vi "Model Initial Values - Remove Inport RTM.vi"(8 "error in (no error)":errorcluster, 11 "Node Ptr":u64 format="%.0x") -> (0 "error out":errorcluster)   [LabVIEW 2011, in "Model Initial Values Custom Device.lvlib"]
uses:
  Model Initial Values Custom Device.lvlib
  <vilib>/NI Veristand/Custom Device API/Custom Device Item Ref.ctl
  NationalInstruments.VeriStand.SystemStorage
  Model Initial Values - Global.vi
  <vilib>/NI Veristand/Custom Device API/Get Item Property (Dependent Node Pointer).vi
  <vilib>/NI Veristand/Custom Device API/Set Item Property (Double Array).vi
  <vilib>/NI Veristand/Custom Device API/Set Item Property (String Array).vi
  <vilib>/NI Veristand/Custom Device Tools/Custom Device Utility Library/Custom Device Utility Library.lvlib
  <vilib>/NI Veristand/Custom Device API/Custom Device API.lvlib
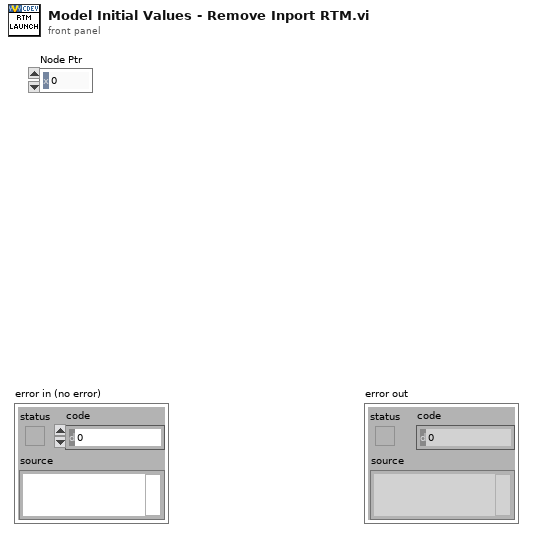
[diagram p1: front panel]
types:
  T1 = typedef "Custom Device API.lvlib/Custom Device Item Ref.ctl" = u64
  T2 = cluster{"MultipleSelection":bool, "ShowCheckBox":bool}
  T3 = typedef "Custom Device API.lvlib/Custom Device Item Info.ctl" = cluster{"Name":string, "Is Channel":bool, "GUID":string}
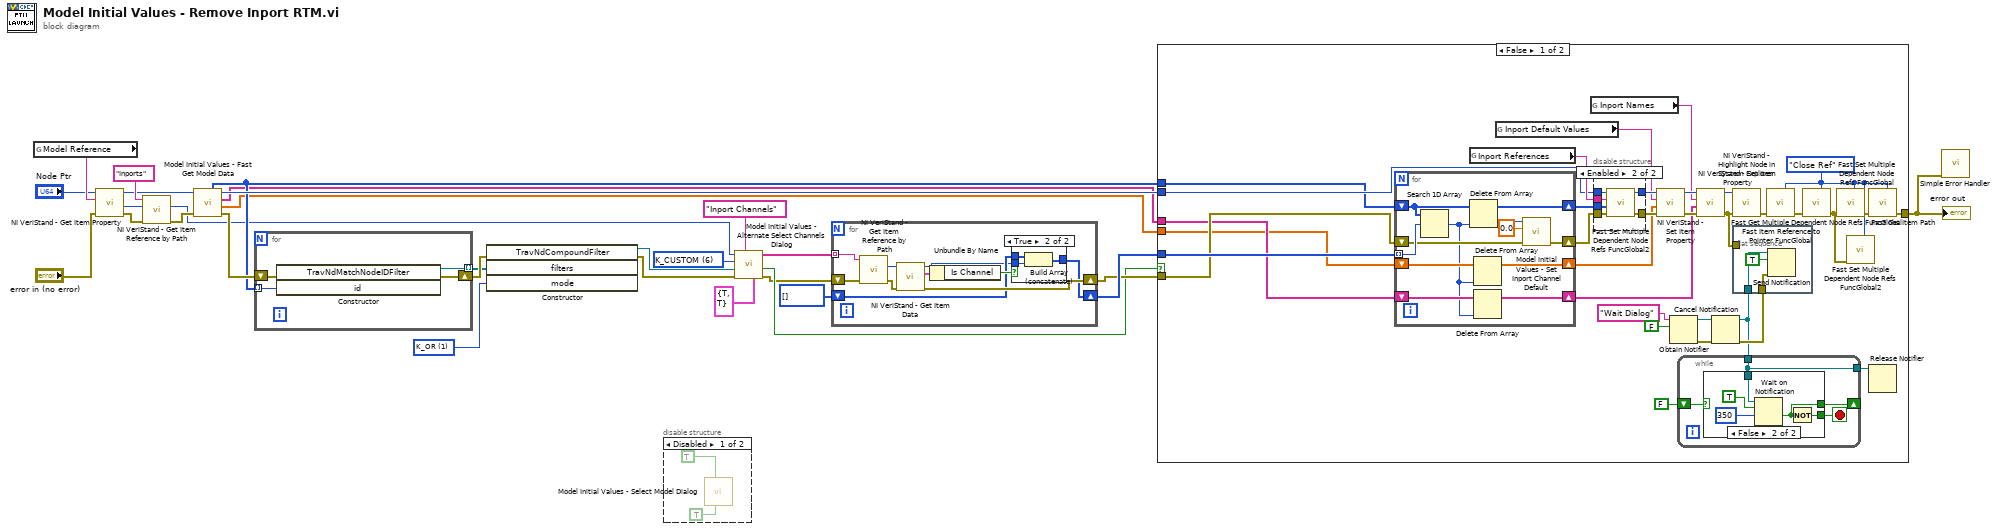
[diagram p0: block diagram]
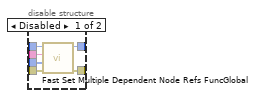
[diagram p4: hidden frame]
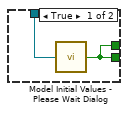
[diagram p5: hidden frame]
diagram:
  w13 = 1 items=["K_AND", "K_OR"] ("mode")
  w18 = u8 6 items=["K_CHAN_R", "K_CHAN_W", "K_CHAN_RW", "K_CHAN_VOLT", "K_CHAN_FAULT", "K_ALL", "K_CUSTOM"] ("Filter")
  n1 = global read "Model Initial Values - Global.vi" "Model Reference"() -> (w9:string)
  n2 = call-poly <vilib>:"NI VeriStand - Get Item Property.vi"("error in (no error)"="error in (no error)", "Property Name"=w9, "Item Ref in"="Node Ptr") -> ("error out"=w3:errorcluster, "Dependent Node Ref"=w4:T1, "Item Ref out"=w6:T1)  [unwired: 5 in, 1 out]
  n3 = call <vilib>:"NI VeriStand - Get Item Reference by Path.vi"("error in (no error)"=w3, "Root Ref"=w4, "Item Path in"="Inports" ("Relative Item Path")) -> ("error out"=w2:errorcluster, "Item Ref"=w1:T1)  [unwired: 5 in, 2 out]
  n4 = call "Model Initial Values - Fast Get Model Data.vi"("error in (no error)"=w2, "Local Model Ref in"=w6) -> ("error out"=w24:errorcluster, "Inport Default Values"=w21:dbl[], "Inport Names"=w22:string[], "Local Model Ref out"=w25:T1, "Inport Refs"=w23:T1[])  [unwired: 4 in, 1 out]
  n5 = for {
    tunnel: [w33] -> w12 mode=indexing
    shift-right: [w32] -> w14
    shift-left: w24 -> [w31]
    tunnel: w23 -> [w30] mode=indexing
    n6 = constructor class="TravNdMatchNodeIDFilter"(error in=w31, "id"=w30) -> (reference out=w33:refnum<k24>, error out=w32:errorcluster)  [unwired: 2 in, 2 out]
  }
  n7 = constructor class="TravNdCompoundFilter"(error in=w14, "filters"=w12, "mode"=w13) -> (reference out=w10:refnum<k24>, error out=w11:errorcluster)  [unwired: 2 in, 3 out]
  n8 = disable-structure shown="Disabled" {
    frame Disabled {
      n9 = call "Model Initial Values - Select Model Dialog.vi"("Multi-Selection?"=TRUE, "References?"=TRUE) -> ()  [unwired: 7 in, 3 out]
    }
    frame Enabled {
    }
  }
  n10 = call "Model Initial Values - Alternate Select Channels Dialog.vi"("Selection Properties"=T2 {"MultipleSelection"=TRUE, "ShowCheckBox"=TRUE}, "Channel Label"="Inport Channels", "error in (no error)"=w11, "Custom Filter"=w10, "Filter"=w18, "Start Item Ref"=w1) -> ("error out"=w15:errorcluster, "Canceled"=w26:bool, "Channel Paths"=w16:string[])  [unwired: 2 in, 1 out]
  n11 = for {
    tunnel: w16 -> [w44] mode=indexing
    shift-right: [w41] -> w27
    shift-left: w15 -> [w45]
    shift-right: [w36] -> w29
    shift-left: T1[] [] -> [w38]
    n12 = call <vilib>:"NI VeriStand - Get Item Reference by Path.vi"("error in (no error)"=w45, "Item Path in"=w44) -> ("error out"=w42:errorcluster, "Item Ref"=w43:T1)  [unwired: 6 in, 2 out]
    n13 = call <vilib>:"NI VeriStand - Get Item Data.vi"("error in (no error)"=w42, "Item Ref in"=w43) -> ("error out"=w41:errorcluster, "Item Info"=w40:T3, "Item Ref out"=w37:T1)  [unwired: 6 in, 1 out]
    n14 = Unbundle By Name(w40) -> ("Is Channel"=w39:bool)
    n15 = case shown="True" w39 {
      tunnel: w38 -> [w46 w49]
      tunnel: w37 -> [_ w48]
      tunnel: [w46 w47] -> w36
      frame False {
      }
      frame True {
        n16 = Build Array (concatenate)(w49, w48) -> (w47:T1[])
      }
    }
  }
  n17 = case shown="False" w26 {
    tunnel: w29 -> [w82 _]
    tunnel: [w56 w121] -> w28
    tunnel: w25 -> [w72 _]
    tunnel: w27 -> [w71 w121]
    tunnel: w23 -> [w55 _]
    tunnel: w22 -> [w54 _]
    tunnel: w21 -> [w53 _]
    frame False {
      w51 = enum16{"Open or Add", "Close Ref"}."Close Ref" ("Action")
      n18 = for {
        tunnel: w82 -> [w120] mode=indexing
        shift-right: [w114] -> w77
        shift-left: w71 -> [w115]
        shift-right: [w118] -> w81
        shift-left: w55 -> [w119]
        shift-right: [w112] -> w73
        shift-left: w53 -> [w113]
        shift-right: [w111] -> w67
        shift-left: w54 -> [w110]
        n19 = Search 1D Array(1D array=w119, element=w120) -> (index of element=w109:i32)  [unwired: 1 in]
        n20 = Delete From Array(array=w119, index=w109) -> (deleted portion=w116:T1, array with subset deleted=w118:T1[])  [unwired: 1 in]
        n21 = Delete From Array(array=w113, index=w109) -> (array with subset deleted=w112:dbl[])  [unwired: 1 in, 1 out]
        n22 = Delete From Array(array=w110, index=w109) -> (array with subset deleted=w111:string[])  [unwired: 1 in, 1 out]
        n23 = call "Model Initial Values - Set Inport Channel Default.vi"("error in"=w115, "Default Value"=0.0, "Item Ref in"=w116) -> ("error out"=w114:errorcluster)  [unwired: 7 in, 1 out]
      }
      n24 = global read "Model Initial Values - Global.vi" "Inport References"() -> (w80:string)
      n25 = global read "Model Initial Values - Global.vi" "Inport Default Values"() -> (w74:string)
      n26 = global read "Model Initial Values - Global.vi" "Inport Names"() -> (w52:string)
      n27 = disable-structure shown="Enabled" {
        disable-tunnel: w81 -> [w88 w90]
        disable-tunnel: w80 -> [w87 w89]
        disable-tunnel: w77 -> [w86 w94]
        disable-tunnel: [w85 w93] -> w76
        disable-tunnel: [w84 w92] -> w75
        disable-tunnel: w72 -> [w83 w91]
        frame Disabled {
          n28 = call "Fast Set Multiple Dependent Node Refs FuncGlobal.vi"("error in (no error)"=w86, "Dependent Node Refs"=w88, "Base Property Name"=w87, "Item Ref in"=w83) -> ("error out"=w85:errorcluster, "Item Ref out"=w84:T1)  [unwired: 6 in]
        }
        frame Enabled {
          n29 = call "Fast Set Multiple Dependent Node Refs FuncGlobal2.vi"("error in (no error)"=w94, "Dependent Node Refs"=w90, "Base Property Name"=w89, "Item Ref in"=w91) -> ("error out"=w93:errorcluster, "Item Ref out"=w92:T1)  [unwired: 6 in]
        }
      }
      n30 = call-poly <vilib>:"NI VeriStand - Set Item Property.vi"("error in (no error)"=w76, "Value"=w73, "Property Name"=w74, "Item Ref in"=w75) -> ("error out"=w70:errorcluster, "Item Ref out"=w69:T1)  [unwired: 5 in, 1 out]
      n31 = Obtain Notifier(name (unnamed)="Wait Dialog", notification data type=FALSE) -> (notifier out=w63:refnum<notifier>, error out=w66:errorcluster)  [unwired: 2 in, 1 out]
      n32 = call-poly <vilib>:"NI VeriStand - Set Item Property.vi"("error in (no error)"=w70, "Value"=w67, "Property Name"=w52, "Item Ref in"=w69) -> ("error out"=w58:errorcluster, "Item Ref out"=w68:T1)  [unwired: 5 in, 1 out]
      n33 = Cancel Notification(0:w63, 3:w66) -> (8:w59:refnum<notifier>, 11:w60:errorcluster)  [unwired: 1 out]
      n34 = while {
        tunnel: w59 -> [w95]
        shift-right: [w96] -> _
        shift-left: FALSE -> [w97]
        tunnel: [w95] -> w65
        stop <- w98 stop-if-true
        n35 = case shown="False" w97 {
          tunnel: [w99 w103] -> w98
          tunnel: w95 -> [w100 w105]
          tunnel: [w99 w101] -> w96
          frame True {
            n36 = call "Model Initial Values - Please Wait Dialog.vi"("notifier out"=w100) -> ("Boolean"=w99:bool)
          }
          frame False {
            n37 = Wait on Notification(notifier=w105, ignore previous (F)=TRUE, timeout in ms (-1)=350) -> (timed out?=w101:bool)  [unwired: 1 in, 3 out]
            n38 = Not(x=w101) -> (.not. x?=w103:bool)
          }
        }
      }
      n39 = call <vilib>:"NI VeriStand - Highlight Node in System Explorer.vi"("error in (no error)"=w58, "Item Ref in"=w68) -> ("error out"=w78:errorcluster)  [unwired: 8 in, 1 out]
      n40 = flat-sequence {
        tunnel: w59 -> [w108]
        tunnel: w60 -> [w107]
        tunnel: w58 -> [_]
        frame #0 {
          n41 = Send Notification(notification=TRUE, notifier=w108, error in (no error)=w107) -> ()  [unwired: 2 out]
        }
      }
      n42 = call "Fast Item Reference to Pointer FuncGlobal.vi"("Action"=w51, "error in (no error)"=w78) -> ("error out"=w79:errorcluster)  [unwired: 6 in, 3 out]
      n43 = call "Fast Get Multiple Dependent Node Refs FuncGlobal.vi"("Action"=w51, "error in (no error)"=w79) -> ("error out"=w50:errorcluster)  [unwired: 7 in, 2 out]
      n44 = call "Fast Set Multiple Dependent Node Refs FuncGlobal.vi"("Action"=w51, "error in (no error)"=w50) -> ("error out"=w57:errorcluster)  [unwired: 8 in, 1 out]
      n45 = call "Fast Set Multiple Dependent Node Refs FuncGlobal2.vi"("Action"=w51, "error in (no error)"=w50) -> ()  [unwired: 8 in, 2 out]
      n46 = call "Fast Get Item Path.vi"("Action"=w51, "error in (no error)"=w57) -> ("error out"=w56:errorcluster)  [unwired: 6 in, 3 out]
      n47 = Release Notifier(notifier=w65) -> ()  [unwired: 2 in, 3 out]
    }
    frame True {
    }
  }
  "error out" <- w28
  n48 = call <vilib>:"Simple Error Handler.vi"("error in (no error)"=w28) -> ()  [unwired: 4 in, 5 out]
